vi "去除无效数据_字符串.vi"(0 "关联成像原理":string[](array[string]), 5 "光源散斑类型":string[](array[string]), 7 "图像类型":string[](array[string]), 9 "重建方法":string[](array[string]), 11 "优化算法":string[](array[string])) -> (4 "关联成像原理最终选择":string, 6 "光源散斑类型最终选择":string, 8 "图像类型最终选择":string, 10 "重建方法最终选择":string, 15 "优化算法最终选择":string)   [LabVIEW 2018]
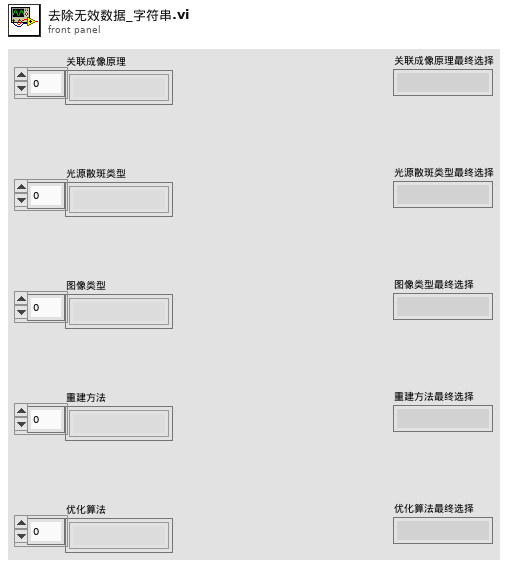
[diagram p1: front panel]
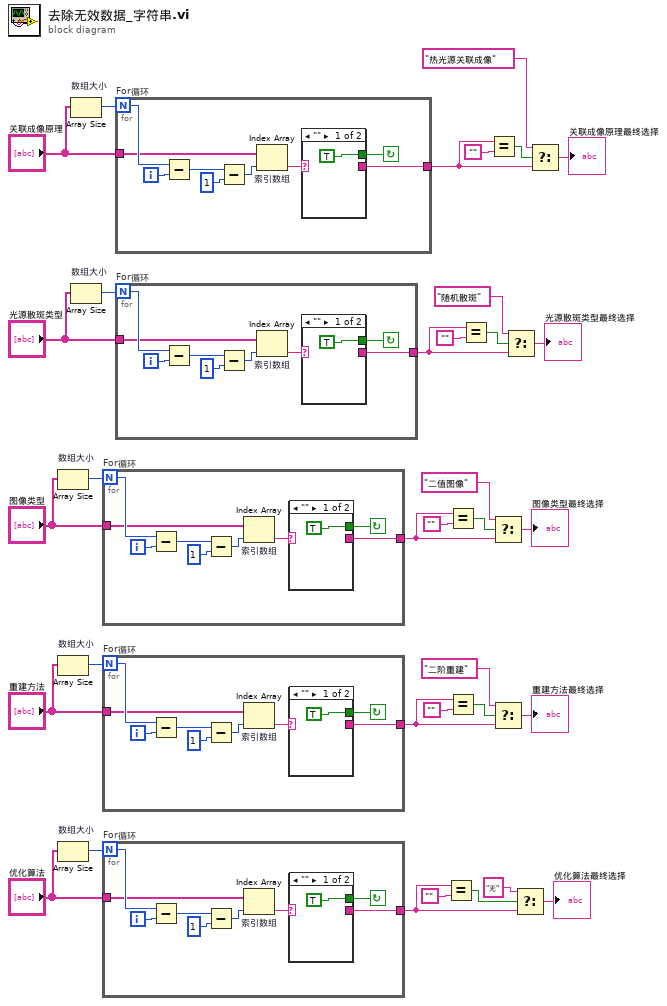
[diagram p0: block diagram]
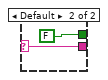
[diagram p2: hidden frame]
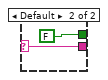
[diagram p3: hidden frame]
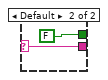
[diagram p4: hidden frame]
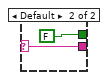
[diagram p5: hidden frame]
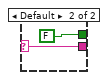
[diagram p6: hidden frame]
diagram:
  n1 = Array Size "数组大小"(array="图像类型") -> (size(s)=w31:i32)
  n2 = Array Size "数组大小"(array="重建方法") -> (size(s)=w29:i32)
  n3 = Array Size "数组大小"(array="优化算法") -> (size(s)=w27:i32)
  n4 = Array Size "数组大小"(array="关联成像原理") -> (size(s)=w35:i32)
  n5 = Array Size "数组大小"(array="光源散斑类型") -> (size(s)=w33:i32)
  n6 = for "For循环" {
    N: w31 -> [w44]
    tunnel: [w37] -> w12
    tunnel: "图像类型" -> [w36]
    i -> [w43]
    stop <- w38 continue-if-true
    n7 = Subtract(x=w44, y=w43) -> (x-y=w42:i32)
    n8 = Subtract(x=w42, y=1) -> (x-y=w40:i32)
    n9 = Index Array "索引数组"(array=w36, index=w40) -> (element=w39:string)
    n10 = case shown="\"\"" w39 {
      selector: w39 -> [_ w46]
      tunnel: [TRUE FALSE] -> w38
      tunnel: [_ w46] -> w37
      frame "" {
      }
      frame Default {
      }
    }
  }
  n11 = for "For循环" {
    N: w29 -> [w56]
    tunnel: [w49] -> w7
    tunnel: "重建方法" -> [w48]
    i -> [w55]
    stop <- w50 continue-if-true
    n12 = Subtract(x=w56, y=w55) -> (x-y=w54:i32)
    n13 = Subtract(x=w54, y=1) -> (x-y=w52:i32)
    n14 = Index Array "索引数组"(array=w48, index=w52) -> (element=w51:string)
    n15 = case shown="\"\"" w51 {
      selector: w51 -> [_ w58]
      tunnel: [TRUE FALSE] -> w50
      tunnel: [_ w58] -> w49
      frame "" {
      }
      frame Default {
      }
    }
  }
  n16 = for "For循环" {
    N: w27 -> [w68]
    tunnel: [w61] -> w2
    tunnel: "优化算法" -> [w60]
    i -> [w67]
    stop <- w62 continue-if-true
    n17 = Subtract(x=w68, y=w67) -> (x-y=w66:i32)
    n18 = Subtract(x=w66, y=1) -> (x-y=w64:i32)
    n19 = Index Array "索引数组"(array=w60, index=w64) -> (element=w63:string)
    n20 = case shown="\"\"" w63 {
      selector: w63 -> [_ w70]
      tunnel: [TRUE FALSE] -> w62
      tunnel: [_ w70] -> w61
      frame "" {
      }
      frame Default {
      }
    }
  }
  n21 = for "For循环" {
    N: w35 -> [w80]
    tunnel: [w73] -> w22
    tunnel: "关联成像原理" -> [w72]
    i -> [w79]
    stop <- w74 continue-if-true
    n22 = Subtract(x=w80, y=w79) -> (x-y=w78:i32)
    n23 = Subtract(x=w78, y=1) -> (x-y=w76:i32)
    n24 = Index Array "索引数组"(array=w72, index=w76) -> (element=w75:string)
    n25 = case shown="\"\"" w75 {
      selector: w75 -> [_ w82]
      tunnel: [TRUE FALSE] -> w74
      tunnel: [_ w82] -> w73
      frame "" {
      }
      frame Default {
      }
    }
  }
  n26 = for "For循环" {
    N: w33 -> [w92]
    tunnel: [w85] -> w17
    tunnel: "光源散斑类型" -> [w84]
    i -> [w91]
    stop <- w86 continue-if-true
    n27 = Subtract(x=w92, y=w91) -> (x-y=w90:i32)
    n28 = Subtract(x=w90, y=1) -> (x-y=w88:i32)
    n29 = Index Array "索引数组"(array=w84, index=w88) -> (element=w87:string)
    n30 = case shown="\"\"" w87 {
      selector: w87 -> [_ w94]
      tunnel: [TRUE FALSE] -> w86
      tunnel: [_ w94] -> w85
      frame "" {
      }
      frame Default {
      }
    }
  }
  n31 = Equal?(x=w2, y="") -> (x = y?=w4:bool)
  n32 = Equal?(x=w12, y="") -> (x = y?=w14:bool)
  n33 = Equal?(x=w7, y="") -> (x = y?=w9:bool)
  n34 = Equal?(x=w17, y="") -> (x = y?=w19:bool)
  n35 = Equal?(x=w22, y="") -> (x = y?=w24:bool)
  n36 = Select(t="二值图像", s=w14, f=w12) -> (s? t:f=→"图像类型最终选择":string)
  n37 = Select(t="二阶重建", s=w9, f=w7) -> (s? t:f=→"重建方法最终选择":string)
  n38 = Select(t="随机散斑", s=w19, f=w17) -> (s? t:f=→"光源散斑类型最终选择":string)
  n39 = Select(t="无", s=w4, f=w2) -> (s? t:f=→"优化算法最终选择":string)
  n40 = Select(t="热光源关联成像", s=w24, f=w22) -> (s? t:f=→"关联成像原理最终选择":string)
